vi "Write Default Headers.vi"(8 "error in (no error)":errorcluster, 10 "Headers":cluster{"header":string, "value":string}[](array[cluster]), 11 "REST Client in":refnum<class "REST Client.lvclass">) -> (0 "error out":errorcluster, 3 "REST Client out":refnum<class "REST Client.lvclass">)   [LabVIEW 2018, in "REST Client_JKI.lvlib" / "REST Client.lvclass"]
doc: "Write Default Headers"
uses:
  REST Client.lvclass
  REST Client.lvclass/REST Client.ctl
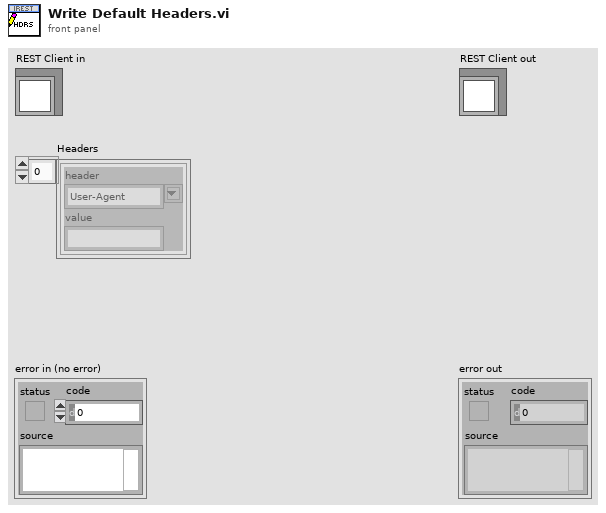
[diagram p1: front panel]
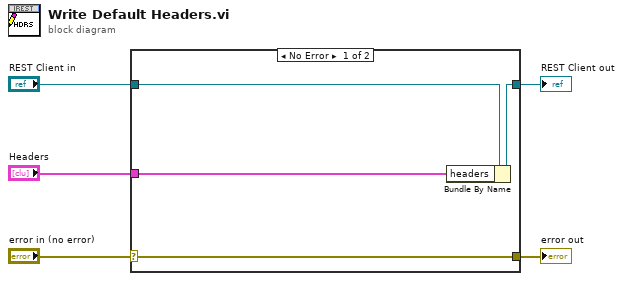
[diagram p0: block diagram]
diagram:
  n1 = case shown="No Error" "error in (no error)" {
    selector: "error in (no error)" -> [w6 w10]
    tunnel: [w6 w10] -> w4
    tunnel: [w9 w11] -> w2
    tunnel: "REST Client in" -> [w7 w11]
    tunnel: "Headers" -> [w8 _]
    frame No Error {
      n2 = Bundle By Name(cluster=w7, "headers"=w8) -> (w9:refnum<class "REST Client.lvclass">)
    }
    frame Error {
    }
  }
  "error out" <- w4
  "REST Client out" <- w2
